vi "TCP-IP.Access.vi"(6 "本地基端口":u16=1120, 7 "IP Address":string="192.168.2.30", 8 "错误输入（无错误）":errorcluster, 9 "CMD":u8[](array[numeric]) format="%02x", 10 "Command":enum16{"Connect", "Read", "Write", "DisConnect"}(ring), 11 "连接ID输入":refnum<k5>) -> (0 "错误输出":errorcluster, 1 "Port":u16, 2 "数据输出":string, 3 "连接ID输出":refnum<k5>)   [LabVIEW 2012, in "Lib_UEL.ATE.lvlib" / "Lib_IPVoice.lvlib"]
uses:
  Lib_IPVoice.lvlib
panel:
  out "remote address 2":string caption="远程地址"
  out "remote port 2":u16 caption="远程端口"
  out "添加的数组":u8[](array[numeric]) format="%02x"
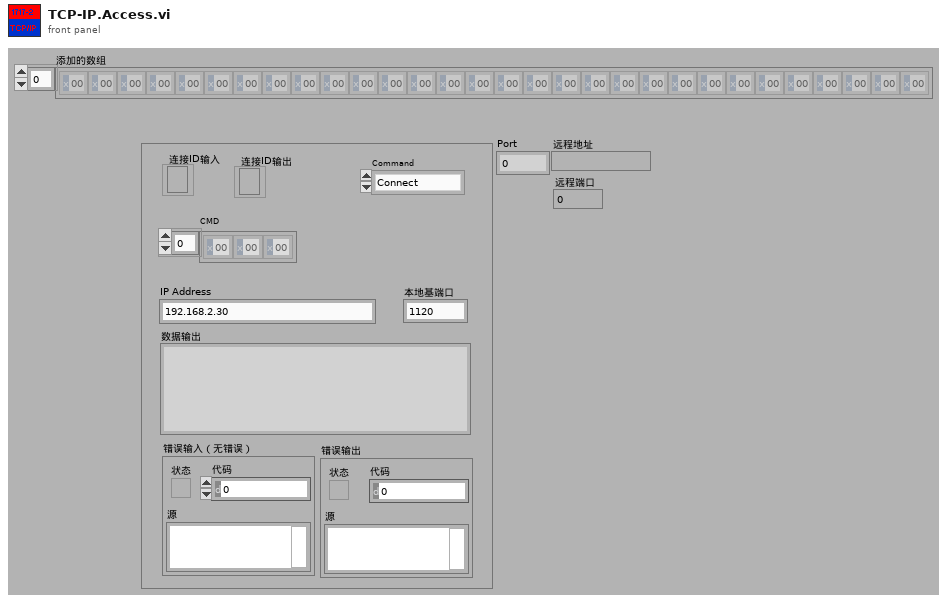
[diagram p1: front panel]
types:
  T1 = enum16{"Standard", "Buffered", "CRLF", "Immediate"}
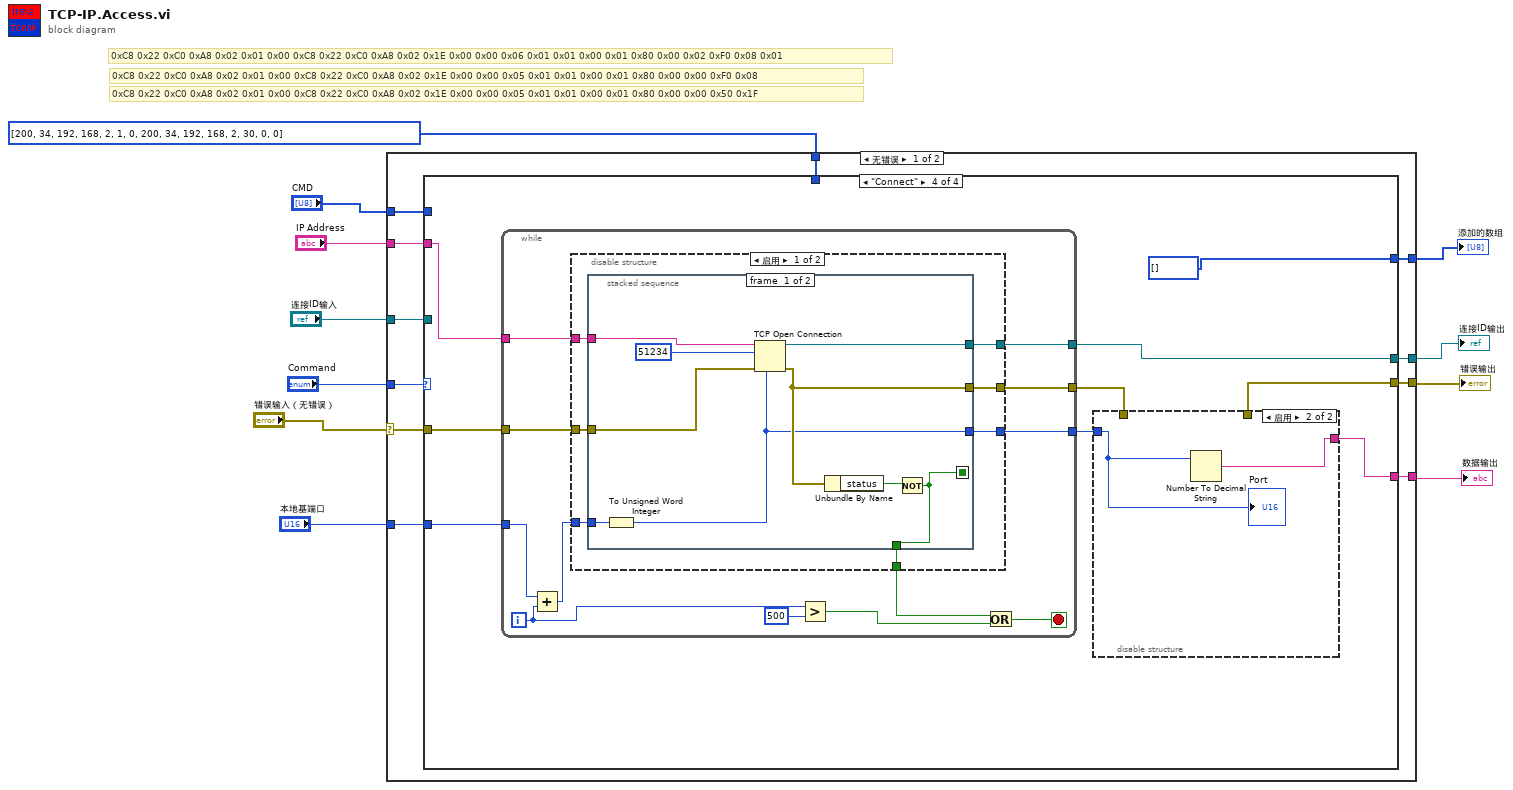
[diagram p0: block diagram]
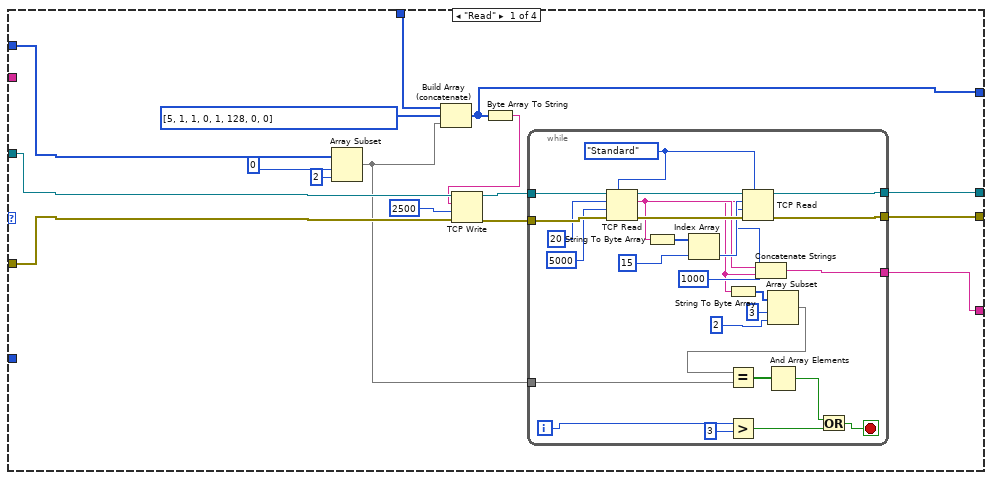
[diagram p2: hidden frame]
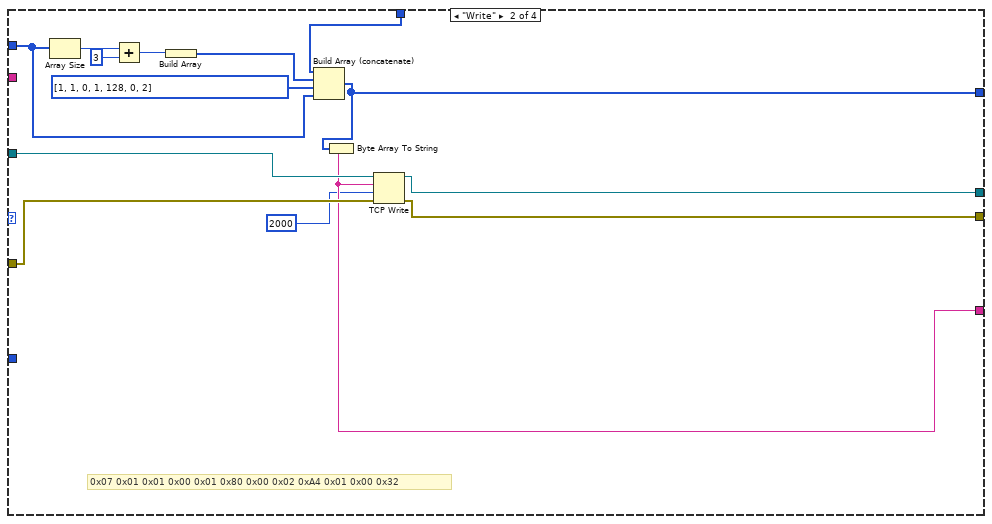
[diagram p3: hidden frame]
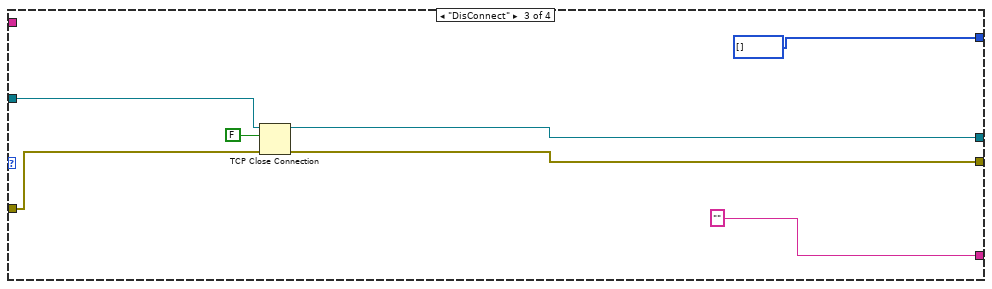
[diagram p4: hidden frame]
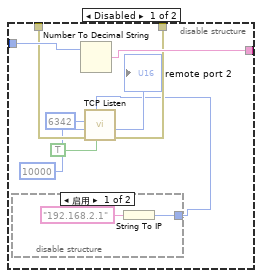
[diagram p5: hidden frame]
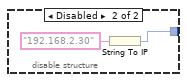
[diagram p6: hidden frame]
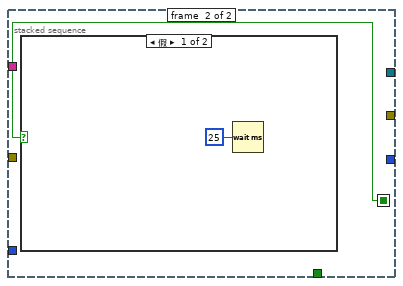
[diagram p7: hidden frame]
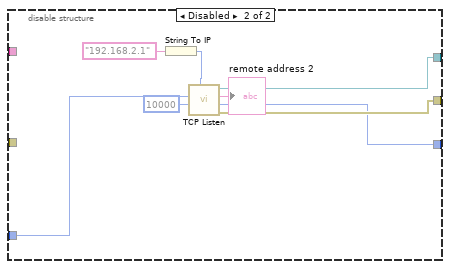
[diagram p9: hidden frame]
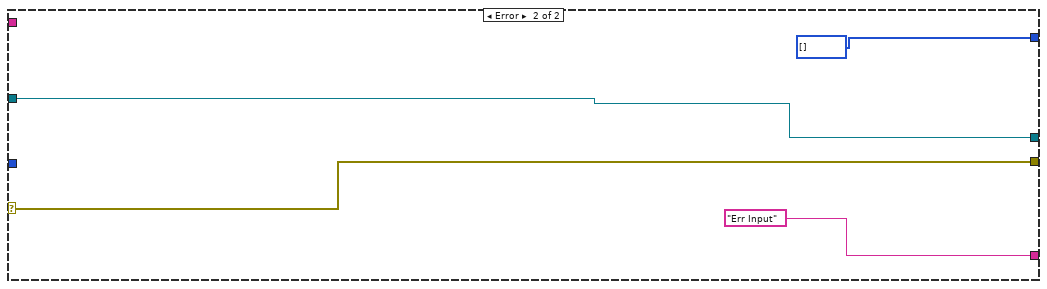
[diagram p10: hidden frame]
diagram:
  # "0xC8 0x22 0xC0 0xA8 0x02 0x01 0x00 0xC8 0x22 0xC0 0xA8 0x02 0x1E 0x00 0x00 0x05 0x01 0x01 0x00 0x01 0x80 0x00 0x00 0x50 0x1F"
  # "0xC8 0x22 0xC0 0xA8 0x02 0x01 0x00 0xC8 0x22 0xC0 0xA8 0x02 0x1E 0x00 0x00 0x05 0x01 0x01 0x00 0x01 0x80 0x00 0x00 0xF0 0x08"
  # "0xC8 0x22 0xC0 0xA8 0x02 0x01 0x00 0xC8 0x22 0xC0 0xA8 0x02 0x1E 0x00 0x00 0x06 0x01 0x01 0x00 0x01 0x80 0x00 0x02 0xF0 0x08 0x01"
  n1 = case shown="无错误" "错误输入（无错误）" {
    selector: "错误输入（无错误）" -> [w17 w151]
    tunnel: "IP Address" -> [w22 _]
    tunnel: "Command" -> [w21 _]
    tunnel: [w20 w151] -> w8
    tunnel: "本地基端口" -> [w19 _]
    tunnel: [w18 w150] -> w6
    tunnel: [w16 "Err Input"] -> w5
    tunnel: "连接ID输入" -> [w15 w150]
    tunnel: "CMD" -> [w14 _]
    tunnel: u8[] [200, 34, 192, 168, 2, 1, 0, 200, 34, 192, 168, 2, 30, 0, 0] ("无符号字节数组") -> [w13 _]
    tunnel: [w12 u8[] []] -> w1
    frame No Error {
      n2 = case shown="\"Connect\"" w21 {
        tunnel: w22 -> [_ _ _ w94]
        tunnel: [w34 w73 w83 w87] -> w20
        tunnel: w19 -> [_ _ _ w95]
        tunnel: [w35 w74 w82 w93] -> w18
        tunnel: w17 -> [w31 w78 w86 w92]
        tunnel: [w36 w75 "" ("string") w90] -> w16
        tunnel: w15 -> [w32 w79 w85 _]
        tunnel: w14 -> [w37 w70 _ _]
        tunnel: w13 -> [w38 w71 _ _]
        tunnel: [w33 w76 u8[] [] u8[] []] -> w12
        frame "Read" {
          n3 = Array Subset(array=w37, index=0 ("索引"), length=2 ("长度")) -> (w23:u8[])
          n4 = Build Array (concatenate)(w38, u8[] [5, 1, 1, 0, 1, 128, 0, 0] ("无符号字节数组"), w23) -> (w33:u8[])
          n5 = Byte Array To String(unsigned byte array=w33) -> (string=w25:string)
          n6 = TCP Write(connection ID=w32, data in=w25, error in (no error)=w31, 9:2500 ("超时毫秒(25000)")) -> (connection ID out=w30:refnum<k5>, error out=w29:errorcluster)  [unwired: 1 out]
          n7 = while {
            tunnel: [w65] -> w36
            tunnel: [w64] -> w35
            tunnel: [w63] -> w34
            tunnel: w30 -> [w62]
            tunnel: w29 -> [w61]
            tunnel: w23 -> [w45]
            i -> [w44]
            stop <- w42 stop-if-true
            w57 = T1."Standard" ("模式（标准）")
            n8 = TCP Read(connection ID=w62, bytes to read=20 ("读取的字节"), error in (no error)=w61, 7:w57, 9:5000 ("超时毫秒(25000)")) -> (connection ID out=w59:refnum<k5>, data out=w53:string, error out=w58:errorcluster)
            n9 = String To Byte Array(string=w53) -> (unsigned byte array=w56:u8[])
            n10 = Index Array(array=w56, index=15 ("索引")) -> (element=w54:u8)
            n11 = Greater?(x=w44, y=3) -> (0:w41:bool)
            n12 = TCP Read(connection ID=w59, bytes to read=w54, error in (no error)=w58, 7:w57, 9:1000 ("超时毫秒(25000)")) -> (connection ID out=w64:refnum<k5>, data out=w50:string, error out=w63:errorcluster)
            n13 = String To Byte Array(string=w50) -> (unsigned byte array=w49:u8[])
            n14 = Concatenate Strings(w53, w50) -> (w65:string)
            n15 = Array Subset(array=w49, index=3 ("索引"), length=2 ("长度")) -> (w46:u8[])
            n16 = Equal?(x=w46, y=w45) -> (x = y?=w40:bool[])
            n17 = And Array Elements(Boolean array=w40) -> (logical AND=w39:bool)
            n18 = Or(x=w39, y=w41) -> (x .or. y?=w42:bool)
          }
        }
        frame "Write" {
          # "0x07 0x01 0x01 0x00 0x01 0x80 0x00 0x02 0xA4 0x01 0x00 0x32"
          n19 = Array Size(array=w70) -> (size(s)=w69:i32)
          n20 = Add(x=w69, y=3) -> (x+y=w67:i32)
          n21 = Build Array(w67) -> (w66:i32[])
          n22 = Build Array (concatenate)(w71, w66, u8[] [1, 1, 0, 1, 128, 0, 2] ("无符号字节数组"), w70) -> (w76:i32[])
          n23 = Byte Array To String(unsigned byte array=w76) -> (string=w75:string)
          n24 = TCP Write(connection ID=w79, data in=w75, error in (no error)=w78, 9:2000 ("超时毫秒(25000)")) -> (connection ID out=w74:refnum<k5>, error out=w73:errorcluster)  [unwired: 1 out]
        }
        frame "DisConnect" {
          n25 = TCP Close Connection(connection ID=w85, abort (F)=FALSE ("中止(F)"), error in (no error)=w86) -> (connection ID out=w82:refnum<k5>, error out=w83:errorcluster)
        }
        frame "Connect" {
          n26 = while {
            tunnel: w95 -> [w120]
            tunnel: w94 -> [w122]
            tunnel: [w121] -> w93
            tunnel: w92 -> [w119]
            tunnel: [w118] -> w88
            tunnel: [w111] -> w89
            i -> [w116]
            stop <- w112 stop-if-true
            n27 = Add(x=w120, y=w116) -> (x+y=w117:i32)
            n28 = disable-structure shown="启用" {
              disable-tunnel: w122 -> [w129 _]
              disable-tunnel: [w128 w143] -> w121
              disable-tunnel: w119 -> [w127 _]
              disable-tunnel: [w126 w144] -> w118
              disable-tunnel: w117 -> [w125 w146]
              disable-tunnel: [w124 _] -> w114
              disable-tunnel: [w123 w142] -> w111
              frame Enabled {
                n29 = stacked-sequence {
                  seq-local: [w132 _] -> [_ w139]
                  tunnel: w129 -> [w130 _]
                  tunnel: [w132 _] -> w124
                  tunnel: [w136 _] -> w128
                  tunnel: w125 -> [w135 _]
                  tunnel: w127 -> [w134 _]
                  tunnel: [w133 _] -> w126
                  tunnel: [w131 _] -> w123
                  frame #0 {
                    n30 = To Unsigned Word Integer(number=w135) -> (unsigned 16bit integer=w131:u16)
                    n31 = TCP Open Connection(address=w130, remote port or service name=u16 51234 ("远程端口"), local port=w131, error in (no error)=w134) -> (connection ID=w136:refnum<k5>, error out=w133:errorcluster)  [unwired: 1 in]
                    n32 = Unbundle By Name(w133) -> ("status"=w137:bool)
                    n33 = Not(x=w137) -> (.not. x?=w132:bool)
                  }
                  frame #1 {
                    n34 = case shown="假" w139 {
                      frame False {
                        n35 = Wait (ms)(milliseconds to wait=u32 25 ("等待时间（毫秒）")) -> ()  [unwired: 1 out]
                      }
                      frame True {
                      }
                    }
                  }
                }
              }
              frame Disabled {
                n36 = String To IP(1:"192.168.2.1" ("名称")) -> (0:w147:u32)
                n37 = call <vilib>:"TCP Listen.vi"("net address"=w147, "timeout ms (wait forever: -1)"=10000, "port"=w146) -> ("error out"=w144:errorcluster, "remote port"=w142:u16, "remote address"=→"remote address 2":string, "connection ID"=w143:refnum<k5>)  [unwired: 4 in, 1 out]
              }
            }
            n38 = Greater?(x=w116, y=500) -> (0:w113:bool)
            n39 = Or(x=w114, y=w113) -> (x .or. y?=w112:bool)
          }
          n40 = disable-structure shown="启用" {
            disable-tunnel: [w104 w110] -> w90
            disable-tunnel: w89 -> [w103 w109]
            disable-tunnel: w88 -> [w102 _]
            disable-tunnel: [w101 _] -> w87
            frame Disabled {
              n41 = disable-structure shown="启用" {
                disable-tunnel: [w106 w107] -> w98
                frame Enabled {
                  n42 = String To IP(1:"192.168.2.1" ("名称")) -> (0:w106:u32)
                }
                frame Disabled {
                  n43 = String To IP(1:"192.168.2.30" ("名称")) -> (0:w107:u32)
                }
              }
              n44 = Number To Decimal String(number=w103) -> (decimal integer string=w104:string)  [unwired: 1 in]
              n45 = call <vilib>:"TCP Listen.vi"("resolve remote address (T)"=TRUE, "net address"=w98, "error in (no error)"=w102, "timeout ms (wait forever: -1)"=10000, "port"=u16 6342) -> ("error out"=w101:errorcluster, "remote port"=→"remote port 2":u16)  [unwired: 2 in, 3 out]
            }
            frame Enabled {
              n46 = Number To Decimal String(number=w109) -> (decimal integer string=w110:string)  [unwired: 1 in]
              "Port" <- w109
            }
          }
        }
      }
    }
    frame Error {
    }
  }
  "错误输出" <- w8
  "连接ID输出" <- w6
  "数据输出" <- w5
  "添加的数组" <- w1
